vi "Configure Pulse (Duty Cycle).vi"(8 "error in (no error)":errorcluster, 10 "Duty Cycle (50 %)":i32=50 min=0 max=100, 11 "VISA resource name":refnum<visa-resource-name>) -> (0 "error out":errorcluster, 3 "VISA resource name out":refnum<visa-resource-name>)   [LabVIEW 2017, in "Keithley 3390.lvlib"]
doc: "Sets the duty cycle of the pulse waveform."
uses:
  Keithley 3390.lvlib
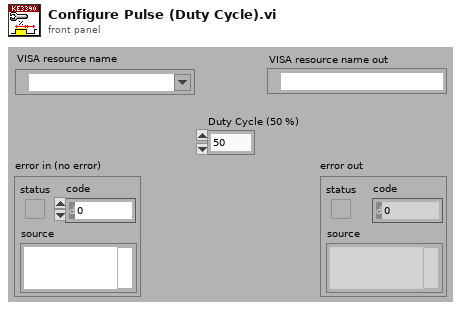
[diagram p1: front panel]
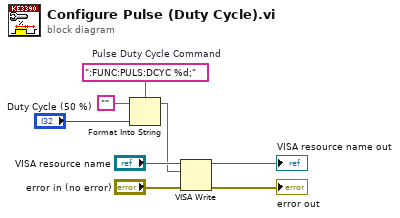
[diagram p0: block diagram]
diagram:
  w6 = ":FUNC:PULS:DCYC %d;"  # Pulse Duty Cycle Command
  n1 = Format Into String(format string=w6, initial string="", "Duty Cycle (50 %)") -> (resulting string=w3:string)  [unwired: 1 in, 1 out]
  n2 = VISA Write(VISA resource name="VISA resource name", write buffer=w3, error in (no error)="error in (no error)") -> (VISA resource name out=→"VISA resource name out":refnum<visa-resource-name>, error out=→"error out":errorcluster)  [unwired: 1 out]
